vi "VISA - Write CMD.vi"(6 "Index":i32, 8 "error in":errorcluster, 9 "Data":T1={"Test"={"Target Load"=0.0, "Target Disp"=0.0, "Rate"=0.0, "Speed"=0.0}, "Sensor"={"Name"=[], "Unit"=[], "Decimal Point"=[], "Ch Log"=[], "H Alarm"=[], "L Alarm"=[], "H Limit"=[], "L Limit"=[], "Filter"=[], "Gain"=[], "Calib Type"=[]}, "PID"={"SP"=0.0, "PV"=0.0, "kP"=0.0, "kI"=0.0, "kD"=0.0, "FF"=0.0, "Err Band"=0.0, "Max"=0, "Min"=0, "Ts"=0, "Out"=0, "Mode"=0}, "ADC"={"Active Ch"=[], "Filter Type"=0, "Post Filter"=[], "Gain"=[], "FS"=0, "IntOC"=0, "IntFC"=0, "SysOC"=0, "Cofficient"=[], "K"=[], "Max"=0}, "System"={"Out Type"=0, "Inverse"=0, "Monitor"=0, "Reserve"=0, "ACC Time"=0, "Pulse Rev"=0, "Stroke"=0, "Auto Off"=0, "Gear Ratio"=0.0, "Pitch"=0.0, "Max Speed"=0, "Jog Speed"=0, "Disp Coff"=0.0, "Max Load"=0}, "Index"=enum."Ch1", "Datalog"=enum."Empty"}, 10 "Action":T2, 11 "VISA ref":refnum<visa-resource-name>) -> (0 "error out":errorcluster, 1 "Data Unit":T3, 2 "Data Channel":T4, 3 "VISA ref out":refnum<visa-resource-name>, 4 "Success":bool, 5 "Bytes at Port":u32, 7 "Prev Data?":bool)   [LabVIEW 2019]
uses:
  Controls/UDP - Command.ctl
  Controls/Communication - Write Data.ctl
  <vilib>/Instr/_visa.llb/VISA Flush IO Buffer Mask.ctl
  Controls/Global - IP Address.vi
  Controls/Global - Handle V1.vi
  Controls/eFGV States.ctl
panel:
  out "x+y":i32
  out "error out 2":errorcluster
  out "appended array":u8[](array[numeric])
  out "*(type *) &x":string
  out "Raw Result":u8[](array[numeric])
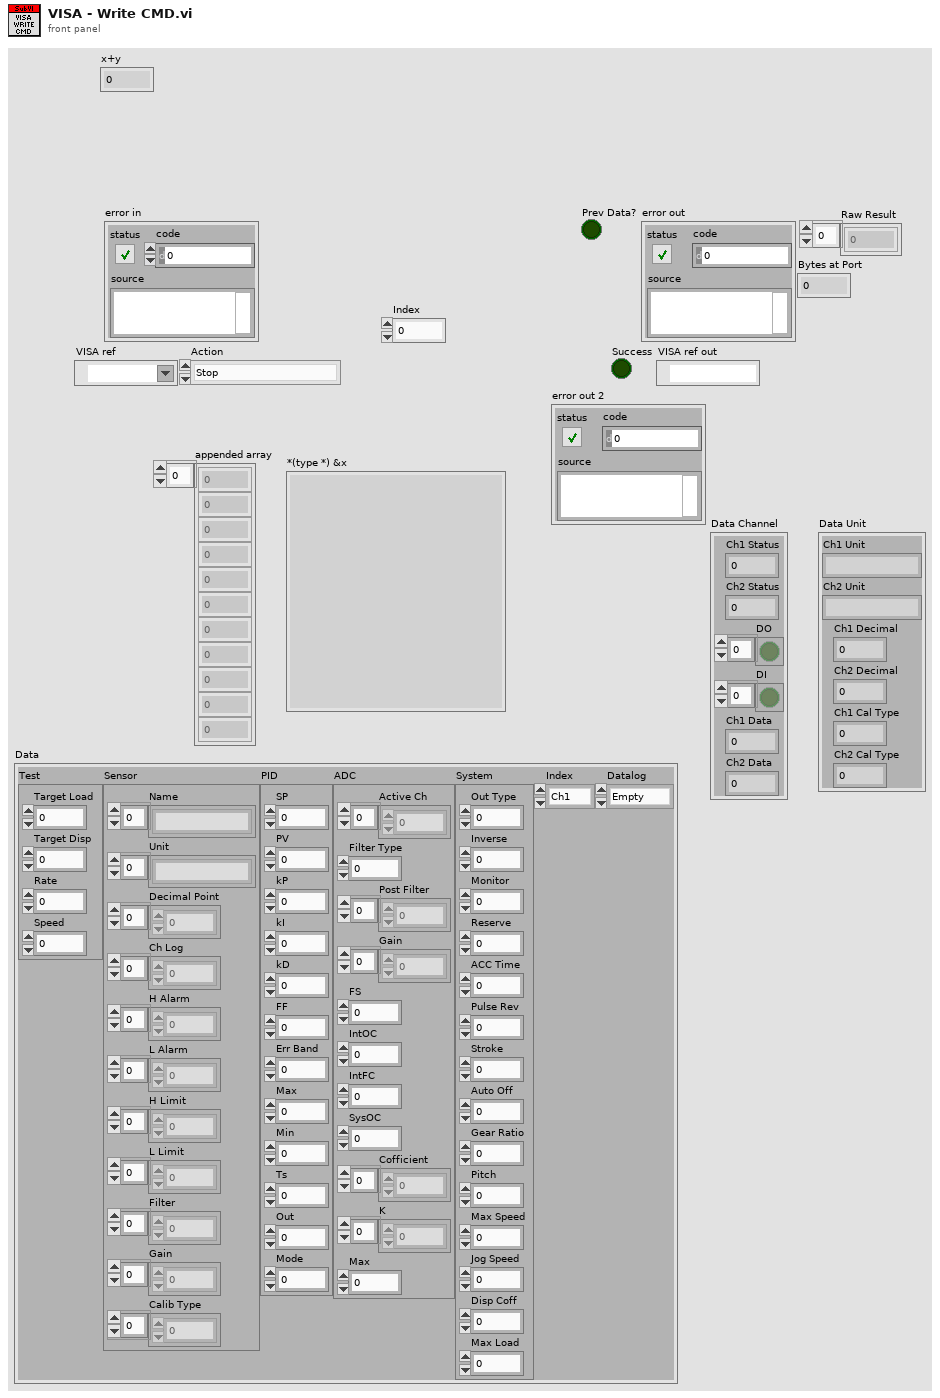
[diagram p1: front panel]
types:
  T1 = typedef "Communication - Write Data.ctl" = cluster{"Test":cluster{"Target Load":sgl, "Target Disp":sgl, "Rate":sgl, "Speed":sgl}, "Sensor":cluster{"Name":string[], "Unit":string[], "Decimal Point":u8[], "Ch Log":u8[], "H Alarm":u8[], "L Alarm":u8[], "H Limit":sgl[], "L Limit":sgl[], "Filter":u8[], "Gain":u8[], "Calib Type":u32[]}, "PID":cluster{"SP":sgl, "PV":sgl, "kP":sgl, "kI":sgl, "kD":sgl, "FF":sgl, "Err Band":sgl, "Max":i32, "Min":i32, "Ts":u32, "Out":i32, "Mode":u8}, "ADC":cluster{"Active Ch":u8[], "Filter Type":u8, "Post Filter":u8[], "Gain":u8[], "FS":u16, "IntOC":u8, "IntFC":u8, "SysOC":u8, "Cofficient":dbl[], "K":dbl[], "Max":i32}, "System":cluster{"Out Type":u8, "Inverse":u8, "Monitor":u8, "Reserve":u8, "ACC Time":u32, "Pulse Rev":u32, "Stroke":u32, "Auto Off":u32, "Gear Ratio":sgl, "Pitch":sgl, "Max Speed":u32, "Jog Speed":u32, "Disp Coff":sgl, "Max Load":u32}, "Index":enum16{"Ch1", "Ch2", "Ch3", "Ch4", "Ch5", "Ch6", "Ch7", "Ch8", "Ch9", "Ch10", "Ch11", "Ch12", "Ch13", "Ch14", "Ch15", "Ch16"}, "Datalog":enum16{"Ch1-Ch16", "Ch17-Ch32", "Ch32-Ch48", "Ch49-Ch64", "Empty"}}
  T2 = typedef "UDP - Command.ctl" = enum16{"Stop", "Jog Up", "Jog Down", "Ramp Up", "Ramp Down", "PID Target", "PID Ramp", "Disp Run", "Read Ch Data", "Zero Channel", "Zero Disp", "Read Sensor", "Write Sensor", "Read ADC", "Write ADC", "Read PID", "Write PID", "Read Test", "Write Test", "Read System", "Write System", "Read Datalog", "Read Datalog Sensor"}
  T3 = cluster{"Ch1 Unit":string, "Ch2 Unit":string, "Ch1 Decimal":u8, "Ch2 Decimal":u8, "Ch1 Cal Type":u8, "Ch2 Cal Type":u8}
  T4 = cluster{"Ch1 Status":u8, "Ch2 Status":u8, "DO":bool[], "DI":bool[], "Ch1 Data":sgl, "Ch2 Data":sgl}
  T5 = typedef "VISA Flush IO Buffer Mask.ctl" = u16
  T6 = typedef "eFGV States.ctl" = enum16{"Init", "Read", "Write", "Exit"}
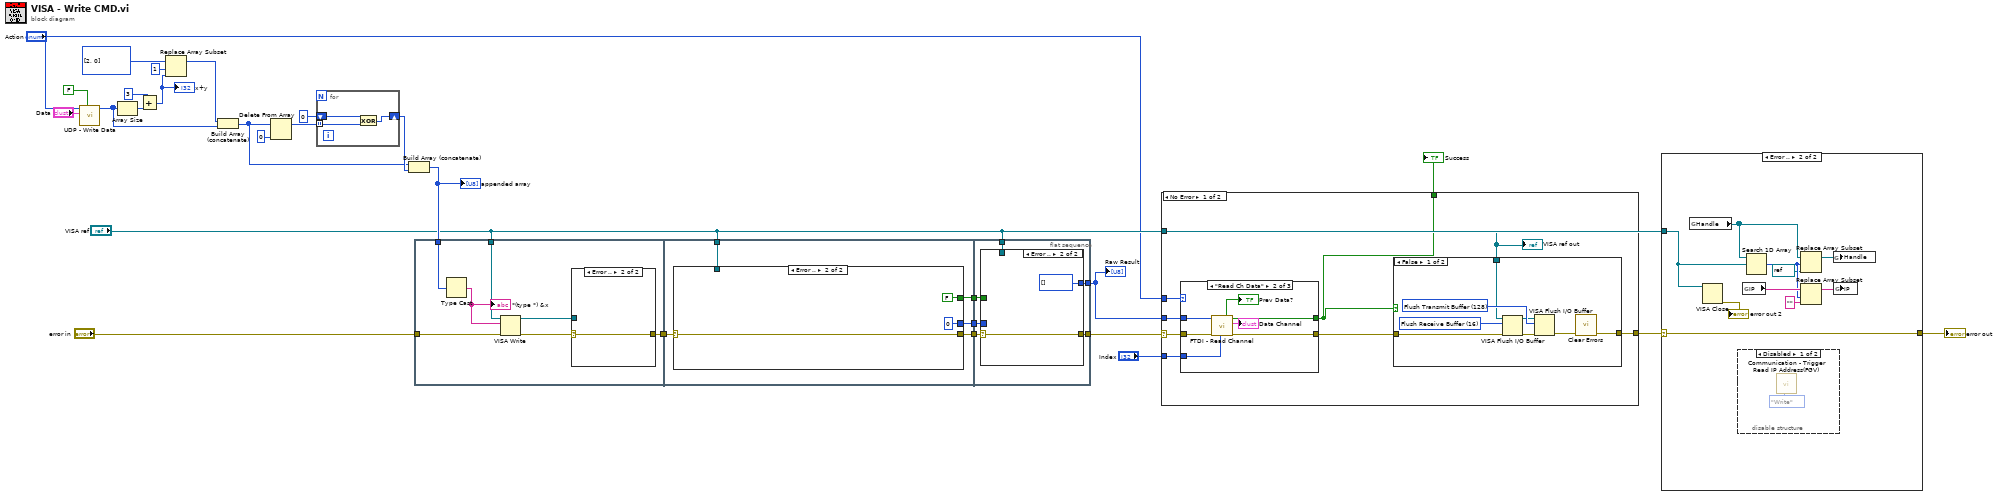
[diagram p0: block diagram]
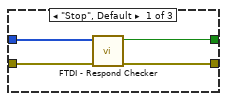
[diagram p3: hidden frame]
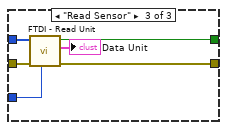
[diagram p4: hidden frame]
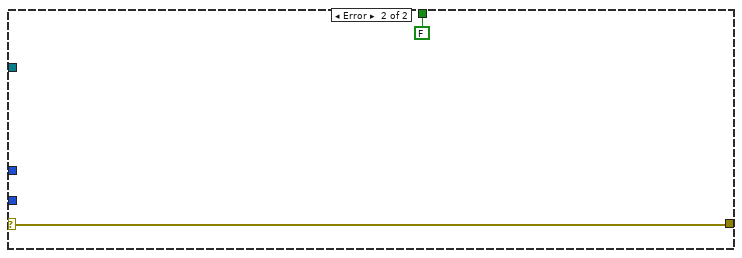
[diagram p5: hidden frame]
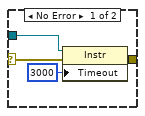
[diagram p8: hidden frame]
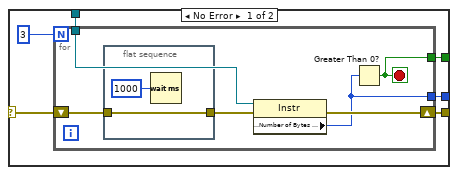
[diagram p9: hidden frame]
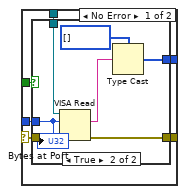
[diagram p10: hidden frame]
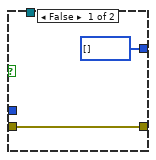
[diagram p11: hidden frame]
diagram:
  n1 = call "UDP - Write Data.vi"("V2"=FALSE, "Data"="Data", "CMD"="Action") -> ("Array"=w15:u8[])  [unwired: 8 in]
  n2 = Array Size(array=w15) -> (size(s)=w11:i32)
  n3 = Add(x=3, y=w11) -> (x+y=w9:i32)
  "x+y" <- w9
  n4 = Replace Array Subset(array=u8[] [2, 0], new element=w9, index=1) -> (w12:u8[])
  n5 = Build Array (concatenate)(w12, w15) -> (w6:u8[])
  n6 = Delete From Array(array=w6, index=0) -> (array with subset deleted=w26:u8[])  [unwired: 1 in, 1 out]
  n7 = for {
    shift-right: [w30] -> w25
    shift-left: u8 0 ("Numeric") -> [w31]
    tunnel: w26 -> [w29] mode=indexing
    n8 = Exclusive Or(1:w29, 2:w31) -> (0:w30:u8)
  }
  n9 = Build Array (concatenate)(w6, w25) -> (w24:u8[])
  "appended array" <- w24
  n10 = flat-sequence {
    tunnel: w24 -> [w36]
    tunnel: [w34] -> w19
    tunnel: "VISA ref" -> [w37]
    tunnel: "error in" -> [w38]
    tunnel: [w48] -> w23
    tunnel: w19 -> [w44]
    tunnel: "VISA ref" -> [w47]
    tunnel: [w46] -> w20
    tunnel: [w45] -> w3
    tunnel: [w69] -> w21
    tunnel: [w71] -> w2
    tunnel: w23 -> [w66]
    tunnel: "VISA ref" -> [w70]
    tunnel: w20 -> [w68]
    tunnel: w3 -> [w67]
    frame #0 {
      n11 = Type Cast(x=w36) -> (*(type *) &x=w35:string)  [unwired: 1 in]
      "*(type *) &x" <- w35
      n12 = VISA Write(VISA resource name=w37, write buffer=w35, error in (no error)=w38) -> (VISA resource name out=w33:refnum<visa-resource-name>, error out=w32:errorcluster)  [unwired: 1 out]
      n13 = case shown="Error .." w32 {
        selector: w32 -> [w39 w43]
        tunnel: [w42 w43] -> w34
        tunnel: w33 -> [w41 _]
        frame No Error {
          n14 = property class="Instr"(reference=w41, error in=w39, "Timeout"=u32 3000 ("General Settings:Timeout Value")) -> (error out=w42:errorcluster)  [unwired: 1 out]
        }
        frame Error {
        }
      }
    }
    frame #1 {
      n15 = case shown="Error .." w44 {
        selector: w44 -> [w49 w65]
        tunnel: [w54 w65] -> w48
        tunnel: w47 -> [w53 _]
        tunnel: [w52 u32 0 ("Bytes at Port")] -> w46
        tunnel: [w50 FALSE] -> w45
        frame No Error {
          n16 = for {
            N: 3 -> [_]
            tunnel: w53 -> [w59]
            tunnel: [w57] -> w52
            shift-right: [w60] -> w54
            shift-left: w49 -> [w55]
            tunnel: [w58] -> w50
            stop <- w58 stop-if-true
            n17 = flat-sequence {
              tunnel: [w61] -> w56
              tunnel: w55 -> [w61]
              frame #0 {
                n18 = Wait (ms)(milliseconds to wait=u32 1000) -> ()  [unwired: 1 out]
              }
            }
            n19 = property class="Instr"(reference=w59, error in=w56) -> (error out=w60:errorcluster, "Serial Settings:Number of Bytes at Serial Port"=w57:u32)  [unwired: 1 out]
            n20 = Greater Than 0?(x=w57) -> (x > 0?=w58:bool)
          }
        }
        frame Error {
        }
      }
    }
    frame #2 {
      n21 = case shown="Error .." w66 {
        selector: w66 -> [w72 w87]
        tunnel: [w77 w87] -> w71
        tunnel: w70 -> [w76 _]
        tunnel: [w75 u8[] [] ("appended array")] -> w69
        tunnel: w68 -> [w74 _]
        tunnel: w67 -> [w73 _]
        frame No Error {
          n22 = case shown="True" w73 {
            tunnel: [w79 w86] -> w77
            tunnel: w72 -> [w79 w85]
            tunnel: w76 -> [_ w84]
            tunnel: w74 -> [_ w83]
            tunnel: [u8[] [] ("appended array") w80] -> w75
            frame False {
            }
            frame True {
              n23 = VISA Read(VISA resource name=w84, byte count=w83, error in (no error)=w85) -> (read buffer=w82:string, error out=w86:errorcluster)  [unwired: 2 out]
              n24 = Type Cast(type=u8[] [] ("appended array"), x=w82) -> (*(type *) &x=w80:u8[])
              "Bytes at Port" <- w83
            }
          }
        }
        frame Error {
        }
      }
    }
  }
  n25 = case shown="No Error" w2 {
    selector: w2 -> [w90 w123]
    tunnel: w21 -> [w96 _]
    tunnel: [w94 w123] -> w18
    tunnel: "VISA ref" -> [w93 _]
    tunnel: "Action" -> [w92 _]
    tunnel: "Index" -> [w91 _]
    tunnel: [w89 FALSE ("Success")] -> w1
    frame No Error {
      n26 = case shown="\"Read Ch Data\"" w92 {
        tunnel: [w108 w115 w118] -> w95
        tunnel: w90 -> [w108 w114 w121]
        tunnel: w96 -> [w107 w113 w120]
        tunnel: [w106 w112 w119] -> w89
        tunnel: w91 -> [_ w110 w116]
        frame "Stop", Default {
          n27 = call "FTDI - Respond Checker.vi"("Read Data"=w107) -> ("Success"=w106:bool)  [unwired: 10 in]
        }
        frame "Read Ch Data" {
          n28 = call "FTDI - Read Channel.vi"("index"=w110, "error in"=w114, "Result"=w113) -> ("error out"=w115:errorcluster, "Data Channel"=→"Data Channel":T4, "Success"=w112:bool, "Prev Data?"=→"Prev Data?":bool)  [unwired: 5 in]
        }
        frame "Read Sensor" {
          n29 = call "FTDI - Read Unit.vi"("Index"=w116, "error in"=w121, "Result"=w120) -> ("error out"=w118:errorcluster, "Data Unit"=→"Data Unit":T3, "Success"=w119:bool)  [unwired: 6 in]
        }
      }
      n30 = case shown="False" w89 {
        tunnel: w95 -> [w100 w105]
        tunnel: [w97 w105] -> w94
        tunnel: w93 -> [w98 _]
        frame False {
          w103 = T5 128 items=["Flush Receive Buffer"=16, "Write Transmit Buffer to Device"=32, "Flush Receive Buffer (No I/O)"=64, "Flush Transmit Buffer"=128] ("Mask")
          w104 = T5 16 items=["Flush Receive Buffer"=16, "Write Transmit Buffer to Device"=32, "Flush Receive Buffer (No I/O)"=64, "Flush Transmit Buffer"=128] ("Mask")
          n31 = VISA Flush I/O Buffer(VISA resource name=w98, mask (16)=w104, error in (no error)=w100) -> (VISA resource name out=w101:refnum<visa-resource-name>, error out=w102:errorcluster)
          n32 = VISA Flush I/O Buffer(VISA resource name=w101, mask (16)=w103, error in (no error)=w102) -> (error out=w99:errorcluster)  [unwired: 1 out]
          n33 = call <vilib>:"Clear Errors.vi"("error in (no error)"=w99) -> ("error out"=w97:errorcluster)  [unwired: 5 in, 1 out]
        }
        frame True {
        }
      }
      "VISA ref out" <- w93
    }
    frame Error {
    }
  }
  "Success" <- w1
  n34 = case shown="Error .." w18 {
    selector: w18 -> [w124 w134]
    tunnel: [w124 w134] -> w17
    tunnel: "VISA ref" -> [_ w126]
    frame No Error {
    }
    frame Error {
      n35 = global read "Global - Handle V1.vi" "Handle"() -> (w133:refnum<visa-resource-name>[])
      n36 = VISA Close(VISA resource name=w126) -> (error out=→"error out 2":errorcluster)  [unwired: 1 in]
      n37 = disable-structure shown="Disabled" {
        frame Disabled {
          n38 = call "Communication - Trigger Read IP Address(FGV).vi"("Action"=eFGV_States."Write") -> ()  [unwired: 8 in, 3 out]
        }
        frame Enabled {
        }
      }
      n39 = global read "Global - IP Address.vi" "IP"() -> (w131:string[])
      n40 = Search 1D Array(1D array=w133, element=w126) -> (index of element=w130:i32)  [unwired: 1 in]
      n41 = Replace Array Subset(array=w133, new element=refnum<visa-resource-name> refnum ("new element/subarray"), index=w130) -> (w132:refnum<visa-resource-name>[])
      n42 = Replace Array Subset(array=w131, new element="" ("new element/subarray"), index=w130) -> (w129:string[])
      n43 = global write "Global - Handle V1.vi" "Handle"(w132) -> ()
      n44 = global write "Global - IP Address.vi" "IP"(w129) -> ()
    }
  }
  "error out" <- w17
  "Raw Result" <- w21
